vi "Get Data.vi"(7 "tdms file":refnum<k34>, 8 "error in (no error)":errorcluster, 11 "GaGe Digitizer in":refnum<class "GaGe Digitizer.lvclass">) -> (0 "error out":errorcluster, 3 "GaGe Digitizer out":refnum<class "GaGe Digitizer.lvclass">)   [LabVIEW 2015, in "GaGe Digitizer.lvclass"]
uses:
  GaGe Digitizer.lvclass
  GaGe Digitizer.lvclass/GaGe Digitizer.ctl
panel:
  out "Data out":waveform(sgl)[](array[waveform])
  in  "First chunk?":bool=TRUE
  in  "Save file?":bool=TRUE
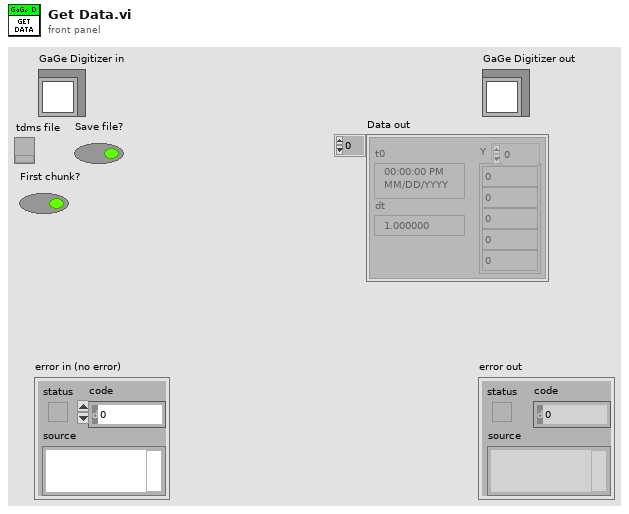
[diagram p1: front panel]
types:
  T1 = cluster{"Handle":u32, "Sample size":u32, "Resolution":i32, "Offset":i32, "Channels":u32, "Boards":u32}
  T2 = cluster{"Device Name":string, "Number of channels":i32, "Device Index":i32, "Device type":enum16{"GaGe", "NI-DAQ", "NI-Scope", "CAMAC", "VXI-1433", "VXI-1437"}, "Total points":i64, "Current position":i64, "Chunk size":i64, "Active":bool, "Oversample by":i32, "Pre-trigger points":i64, "Fast mode":bool}
  T3 = cluster{"Range":dbl, "Coupling":enum16{"Single", "Differen"}, "Impedance":dbl}[]
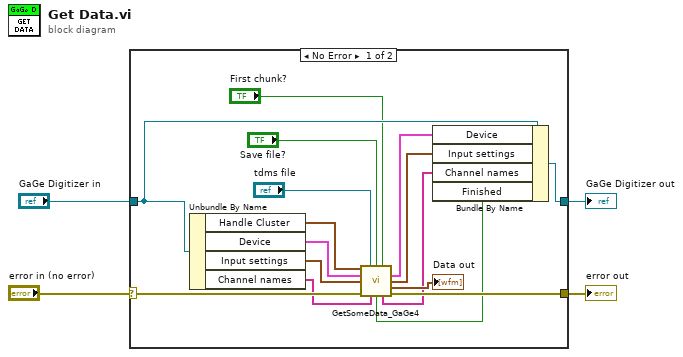
[diagram p0: block diagram]
diagram:
  n1 = case shown="No Error" "error in (no error)" {
    selector: "error in (no error)" -> [w16 w22]
    tunnel: [w15 w22] -> w3
    tunnel: [w10 w21] -> w1
    tunnel: "GaGe Digitizer in" -> [w20 w21]
    frame No Error {
      n2 = Unbundle By Name(w20) -> ("Handle Cluster"=w19:T1, "Device"=w18:T2, "Input settings"=w17:T3, "Channel names"=w14:string[])
      n3 = call "GetSomeData_GaGe4.vi"("Handle Cluster"=w19, "tdms file"="tdms file", "Save file?"="Save file?", "First chunk?"="First chunk?", "Device"=w18, "Input settings"=w17, "error in (no error)"=w16, "Channel names in"=w14) -> ("Device out"=w9:T2, "Input settings out"=w5:T3, "Data out"=→"Data out":waveform(sgl)[], "Finished"=w7:bool, "Channel names out"=w6:string[], "error out"=w15:errorcluster)  [unwired: 2 in]
      n4 = Bundle By Name(cluster=w20, "Device"=w9, "Input settings"=w5, "Channel names"=w6, "Finished"=w7) -> (w10:refnum<class "GaGe Digitizer.lvclass">)
    }
    frame Error {
    }
  }
  "error out" <- w3
  "GaGe Digitizer out" <- w1
